vi "Area de un triangulo.vi"() -> ()   [LabVIEW 2020]
panel:
  out "Area":dbl(knob) scale=0.0..200.0
  in  "Altura":dbl(slide) scale=0.0..60.0
  in  "Base":dbl(slide) scale=0.0..60.0
  # "Area de un trinagulo"
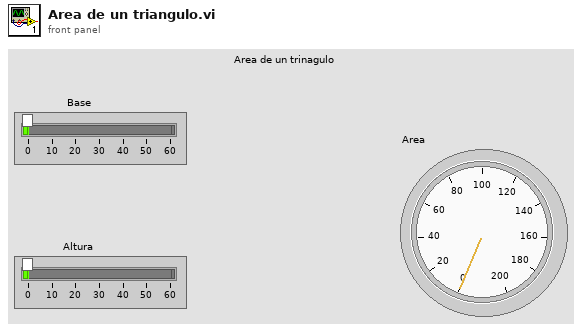
[diagram p1: front panel]
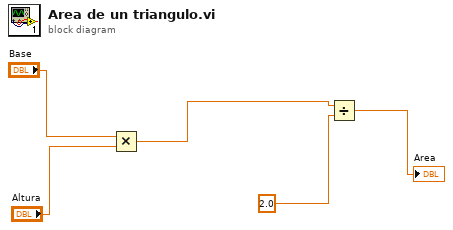
[diagram p0: block diagram]
diagram:
  n1 = Multiply(x="Base", y="Altura") -> (x*y=w3:dbl)
  n2 = Divide(x=w3, y=2.0) -> (x/y=→"Area":dbl)
